vi "pinvTruncate.vi"(9 "Truncation Threshold":dbl=0.0001, 11 "Matrix A":dbl[][](array[numeric])) -> (3 "Truncated Pinv A":dbl[][](array[numeric]))   [LabVIEW 2016]
doc: "Do the pseudo inverse with the truncation based on the threshold."
uses:
  <vilib>/Analysis/baseanly.llb/Real A x B.vi
  <vilib>/Analysis/Matrix/Numeric/Conversions/Array To Matrix - RA2.vi
  <vilib>/Analysis/7linalg.llb/Real SVD Decomposition.vi
  <vilib>/Analysis/Matrix/Numeric/Conversions/Matrix To Array - RM.vi
  <vilib>/Analysis/NI_AALPro.lvlib
  <vilib>/Analysis/NI_AALBase.lvlib
  <vilib>/Analysis/Matrix/NI_Matrix.lvlib
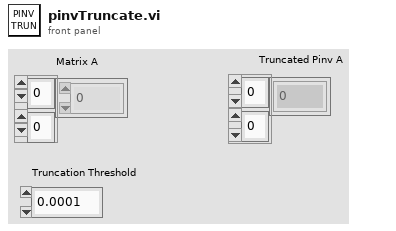
[diagram p1: front panel]
types:
  T1 = typedef "NI_Matrix.lvlib/RealMatrix.ctl" = dbl[][]
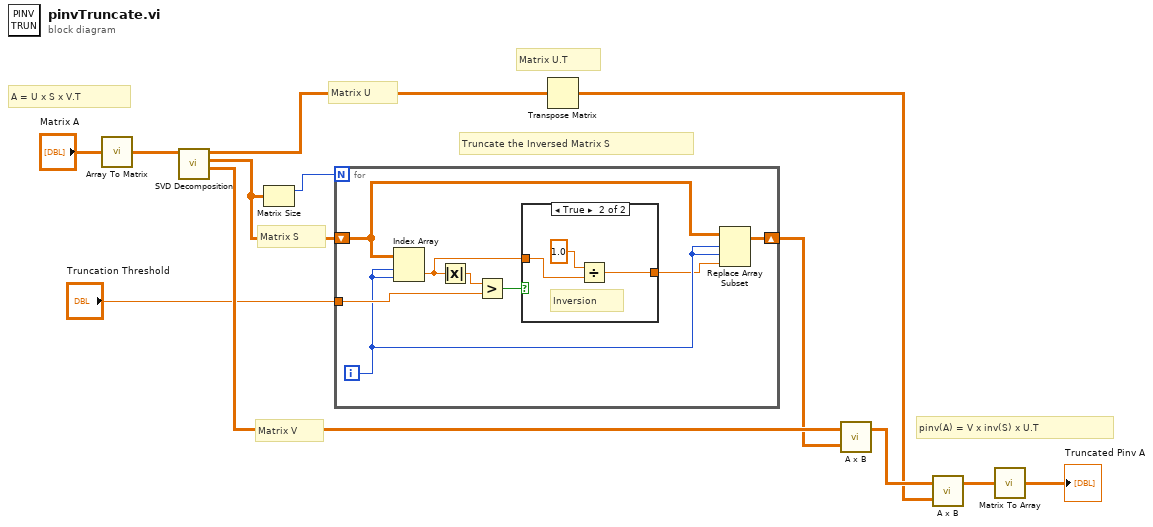
[diagram p0: block diagram]
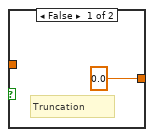
[diagram p2: hidden frame]
diagram:
  # "pinv(A) = V x inv(S) x U.T"
  # "A = U x S x V.T"
  # "Matrix U"
  # "Matrix S"
  # "Truncate the Inversed Matrix S"
  # "Matrix U.T"
  # "Matrix V"
  n1 = call-poly <vilib>:"Array To Matrix.vi"("Real 2D Array"="Matrix A") -> ("Real Matrix"=w11:T1)
  n2 = call-poly <vilib>:"SVD Decomposition.vi"("A"=w11) -> ("Matrix V"=w10:T1, "Matrix S"=w4:T1, "Matrix U"=w8:T1)  [unwired: 6 in, 2 out]
  n3 = Matrix Size(0:w4) -> (1:w6:i32)  [unwired: 1 out]
  n4 = for {
    N: w6 -> [_]
    tunnel: "Truncation Threshold" -> [w19]
    shift-right: [w13] -> w3
    shift-left: w4 -> [w14]
    i -> [w16]
    n5 = Index Array(array=w14, index (row)=w16, index (col)=w16) -> (element=w17:dbl)
    n6 = Absolute Value(x=w17) -> (abs(x)=w20:dbl)
    n7 = Greater?(x=w20, y=w19) -> (0:w18:bool)
    n8 = case shown="True" w18 {
      tunnel: w17 -> [_ w23]
      tunnel: [0.0 w22] -> w15
      frame False {
        # "Truncation"
      }
      frame True {
        # "Inversion"
        n9 = Divide(x=1.0, y=w23) -> (x/y=w22:dbl)
      }
    }
    n10 = Replace Array Subset(array=w14, new element=w15, index (row)=w16, index (col)=w16) -> (w13:T1)
  }
  n11 = Transpose Matrix(1:w8) -> (0:w7:T1)
  n12 = call-poly <vilib>:"A x B.vi"("B"=w3, "A"=w10) -> ("A x B"=w9:T1)  [unwired: 1 out]
  n13 = call-poly <vilib>:"A x B.vi"("B"=w7, "A"=w9) -> ("A x B"=w2:T1)  [unwired: 1 out]
  n14 = call-poly <vilib>:"Matrix To Array.vi"("Real Matrix"=w2) -> ("Real 2D Array"=→"Truncated Pinv A":dbl[][])
